vi "PCO_GetIntensifiedLoopCount.vi"(8 "error in (no error)":errorcluster {"code" format="%x"}, 11 "ph":u64) -> (0 "error out":errorcluster {"code" format="%x"}, 1 "wIntensifiedLoopCount":u16, 2 "ErrorMessage":i32 format="%x", 3 "ph out":u64)   [LabVIEW 2020, in "SDK.lvlib" / "SpecialCommandsDicam.lvlib"]
doc: "SC2_SDK_FUNC int WINAPI PCO_GetIntensifiedLoopCount(HANDLE hCam, WORD *wIntensifiedLoopCount, WORD *wReserved);"
uses:
  SpecialCommandsDicam.lvlib
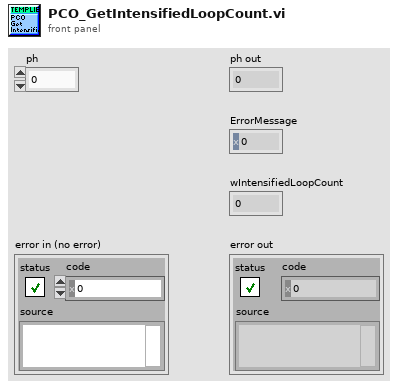
[diagram p1: front panel]
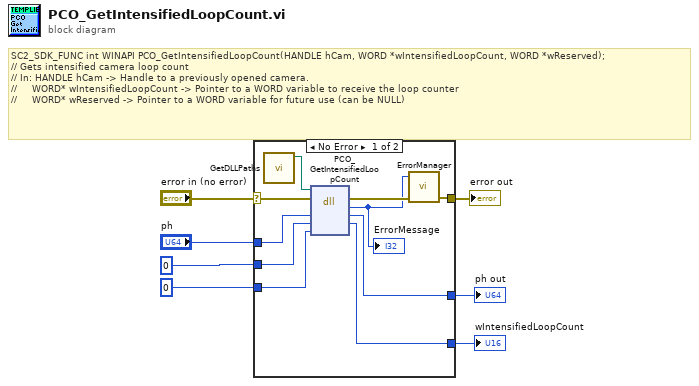
[diagram p0: block diagram]
diagram:
  # "SC2_SDK_FUNC int WINAPI PCO_GetIntensifiedLoopCount(HANDLE hCam, WORD *wIntensifiedLoopCount, WORD *wReserved);\n// Gets intensified camera loop count\n// In: HANDLE hCam -> Handle to a previously opened camera.\n//     WORD* wIntensifiedLoopCount -> Pointer to a WORD variable to receive the loop counter\n//     WORD* wReserved -> Pointer to a WORD variable for future use (can be NULL)"
  n1 = case shown="No Error" "error in (no error)" {
    selector: "error in (no error)" -> [w12 w20]
    tunnel: "ph" -> [w17 w19]
    tunnel: [w16 w19] -> w6
    tunnel: u16 0 ("wIntensifiedLoopCount") -> [w15 w18]
    tunnel: [w14 w18] -> w4
    tunnel: u16 0 ("wReserved") -> [w13 _]
    tunnel: [w11 w20] -> w2
    frame No Error {
      n2 = call "GetDLLPaths.vi"() -> ("SC2_Cam_Path"=w8:path)  [unwired: 9 in, 2 out]
      n3 = dll-call lib="?" fn="PCO_GetIntensifiedLoopCount"(path in=w8, error in=w12, "ph"=w17, "wIntensifiedLoopCount"=w15, "wReserved"=w13) -> (error out=w10:errorcluster, "return type"=w9:i32, "ph"=w16:u64, "wIntensifiedLoopCount"=w14:u16)  [unwired: 2 in, 1 out]
      "ErrorMessage" <- w9
      n4 = call "ErrorManager.vi"("error in (no error)"=w10, "error code"=w9) -> ("error out"=w11:errorcluster)  [unwired: 3 in]
    }
    frame Error {
    }
  }
  "ph out" <- w6
  "wIntensifiedLoopCount" <- w4
  "error out" <- w2
